vi "GaiaActionDelecation.vi"(6 "plainText":string, 8 "Error in":errorcluster, 9 "Action":string, 10 "Application":string, 11 "ClientRef":refnum<k24>) -> (0 "error out":errorcluster, 3 "ClientRef out":refnum<k24>)   [LabVIEW 2018]
uses:
  C:/GIT/gaialabviewclient/Gaia_LabVIEW/Resources/JOT.GaiaClient.dll
  Gaia_LabVIEW/Resources/JOT.GaiaClient.dll
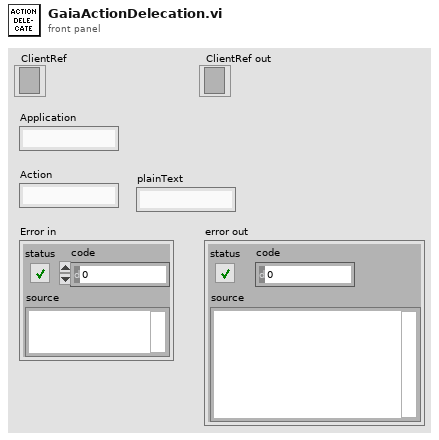
[diagram p1: front panel]
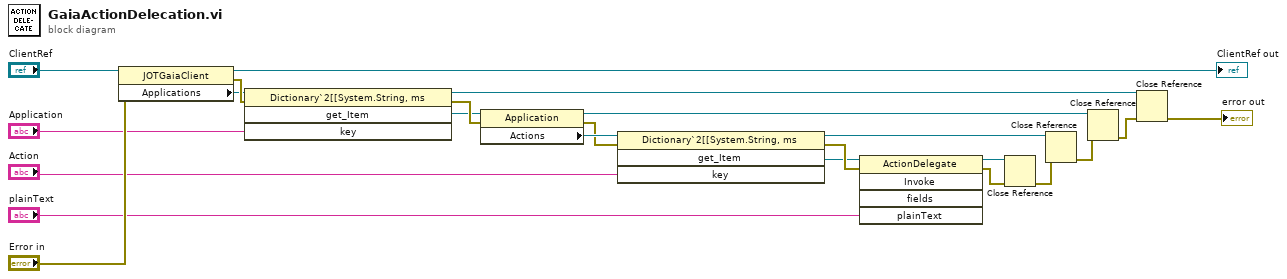
[diagram p0: block diagram]
diagram:
  n1 = property class="JOTGaiaClient"(reference="ClientRef", error in="Error in") -> (reference out=→"ClientRef out":refnum<k24>, error out=w22:errorcluster, "Applications"=w16:refnum<k24>)
  n2 = invoke class="Dictionary`2[[System.String, ms" method="get_Item"(reference=w16, error in=w22, "key"="Application") -> (reference out=w19:refnum<k24>, error out=w8:errorcluster, "get_Item"=w7:refnum<k24>)  [unwired: 1 in, 1 out]
  n3 = property class="Application"(reference=w7, error in=w8) -> (reference out=w12:refnum<k24>, error out=w6:errorcluster, "Actions"=w15:refnum<k24>)
  n4 = invoke class="Dictionary`2[[System.String, ms" method="get_Item"(reference=w15, error in=w6, "key"="Action") -> (reference out=w3:refnum<k24>, error out=w5:errorcluster, "get_Item"=w1:refnum<k24>)  [unwired: 1 in, 1 out]
  n5 = invoke class="ActionDelegate" method="Invoke"(reference=w1, error in=w5, "plainText"="plainText") -> (reference out=w9:refnum<k24>, error out=w4:errorcluster)  [unwired: 2 in, 3 out]
  n6 = Close Reference(reference=w9, error in (no error)=w4) -> (error out=w10:errorcluster)
  n7 = Close Reference(reference=w3, error in (no error)=w10) -> (error out=w11:errorcluster)
  n8 = Close Reference(reference=w12, error in (no error)=w11) -> (error out=w20:errorcluster)
  n9 = Close Reference(reference=w19, error in (no error)=w20) -> (error out=→"error out":errorcluster)
